vi "Select user objective.vi"(8 "error in (no error)":errorcluster, 11 "User objective":string) -> (0 "error out":errorcluster)   [LabVIEW 2020]
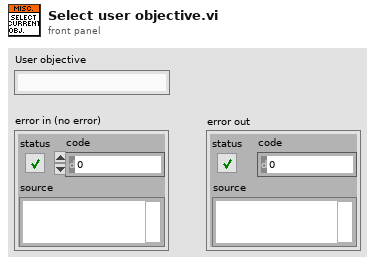
[diagram p1: front panel]
types:
  T1 = enum16{"Init", "Update Objectives", "Update Current Objective", "Read", "Clear"}
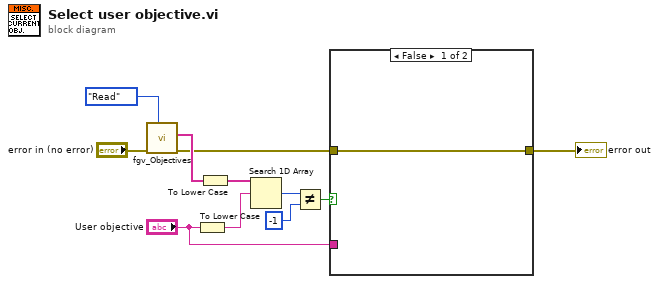
[diagram p0: block diagram]
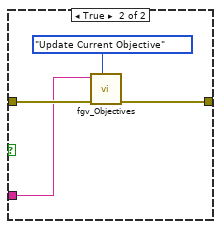
[diagram p2: hidden frame]
diagram:
  n1 = call "fgv_Objectives.vi"("Actions"=T1."Read", "error in (no error)"="error in (no error)") -> ("error out"=w4:errorcluster, "Objectives"=w10:string[])  [unwired: 7 in, 1 out]
  n2 = To Lower Case(string="User objective") -> (all lower case string=w8:string)
  n3 = To Lower Case(string=w10) -> (all lower case string=w9:string[])
  n4 = Search 1D Array(1D array=w9, element=w8) -> (index of element=w7:i32)  [unwired: 1 in]
  n5 = Not Equal?(x=w7, y=-1) -> (x != y?=w5:bool)
  n6 = case shown="False" w5 {
    tunnel: w4 -> [w12 w15]
    tunnel: [w12 w14] -> w2
    tunnel: "User objective" -> [_ w13]
    frame False {
    }
    frame True {
      n7 = call "fgv_Objectives.vi"("Actions"=T1."Update Current Objective", "error in (no error)"=w15, "Current Objective"=w13) -> ("error out"=w14:errorcluster)  [unwired: 6 in, 2 out]
    }
  }
  "error out" <- w2
